vi "Data Processing for cont acq.vi"(4 "error in (no error)":errorcluster, 5 "scan parameters":T1={"scan rate\n(1000 scans/sec)"=1000.0, "scans to read\nat a time (1000)"=1000} {"scan rate\n(1000 scans/sec)" format="%.2f"}, 6 "waveform":waveform(dbl)[](array[waveform]), 7 "voltage data":sgl[][](array[numeric]) format="%.2f") -> (0 "error out":errorcluster, 1 "Intensity Graph":sgl[][](graph), 2 "processed waveform":waveform(dbl)[](array[waveform]), 3 "processed data":sgl[][](array[numeric]) format="%.2f")   [LabVIEW 2022 SP3]
doc: "My Data Processing is a subVI called by some of the analog input example VIs. These examples show you how to process and display data while an acquisition is in progress. This VI is a placeholder to show you where data processing, if any, should be done. Add whatever functions you need to its diagram. You may select Save As from the File menu to save the VI with a more meaningful name, but you should do this when all calling VIs (for example, Acquire & Process N Scans and Acquire & Proc N Scans - Trig) are open, so they are also aware of the name change. Otherwise, you must replace the subVI on each block diagram that uses the old name.\n\nThe processed data array is returned to the example VI to be displayed.\n\nError in is a cluster that indicates if an error has occurred. If so, this VI does not try to process the data, it just returns the voltage data and error unchanged. If an error occurs in your data processing, you should set the following values in the error out cluster:\n\n (bool) status: TRUE.\n\n (i32) code: the error code associated with an error.\n A value of 0 means no error, a negative value is an error,\n and a positive value is a warning.\n\n (string) source: an indication of where the \n error occurred, usually the name of the VI."
uses:
  <vilib>/Waveform/WDTOps.llb/WDT Index Channel DBL.vi
panel:
  in  "Error?":bool
  in  "Case Constant\n(See Context Help)":bool=TRUE
  in  "change window parameters ?":bool
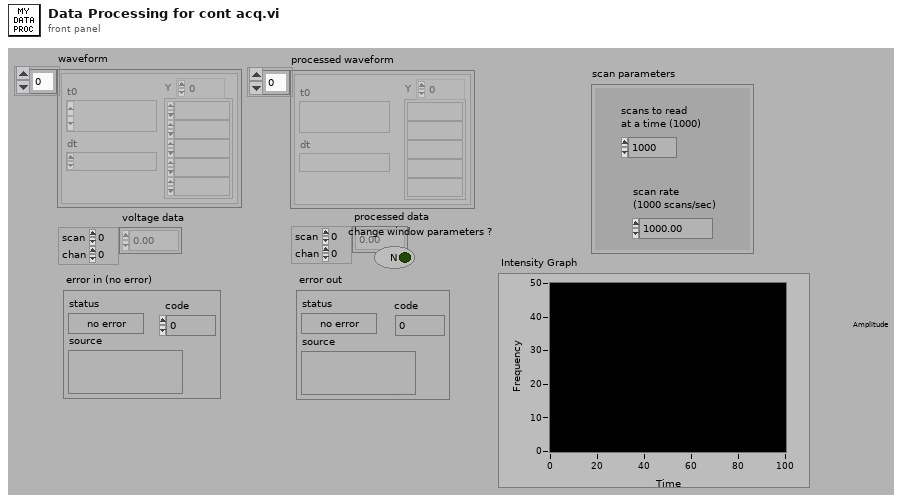
[diagram p1: front panel]
types:
  T1 = cluster{"scan rate\n(1000 scans/sec)":sgl, "scans to read\nat a time (1000)":i32}
  T2 = cluster{"scans to read\nat a time (1000)":i32, "scan rate\n(1000 scans/sec)":sgl, sgl[][]}
  T3 = cluster{"total time slices":i32, "f0":dbl, "Df":dbl, "Dt":dbl}
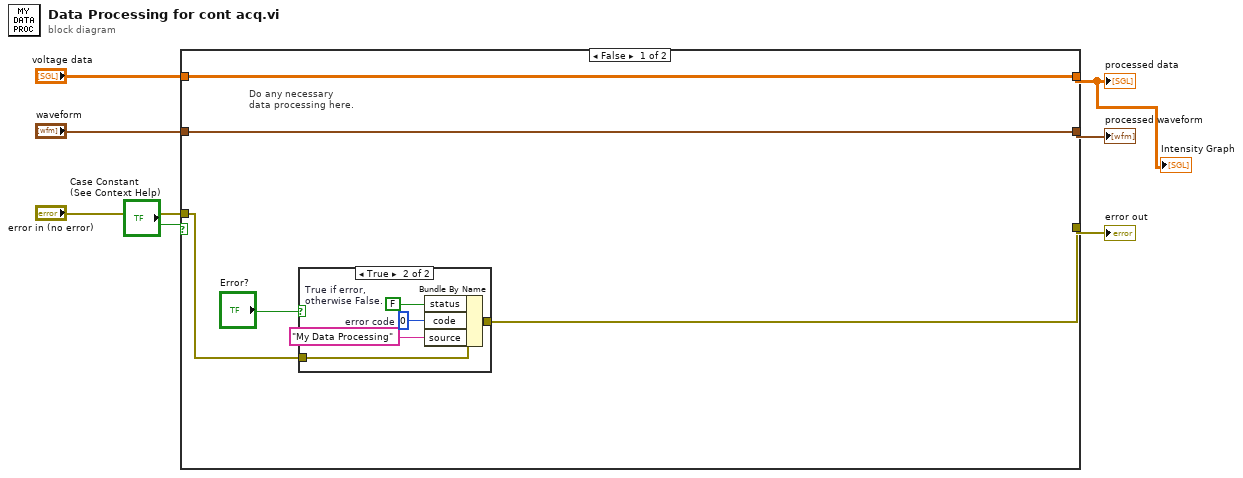
[diagram p0: block diagram]
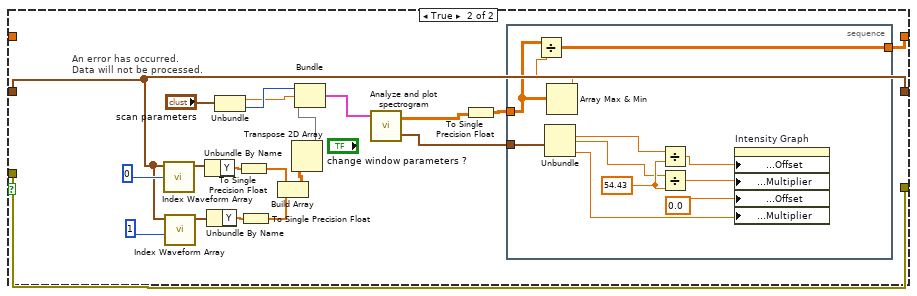
[diagram p3: hidden frame]
diagram:
  n1 = case shown="False" "Case Constant\n(See Context Help)" {
    tunnel: "error in (no error)" -> [w10 w38]
    tunnel: [w9 w38] -> w7
    tunnel: "voltage data" -> [w12 _]
    tunnel: [w12 w19] -> w3
    tunnel: "waveform" -> [w8 w27]
    tunnel: [w8 w27] -> w4
    frame False {
      # "Do any necessary\ndata processing here."
      n2 = case shown="True" "Error?" {
        tunnel: w10 -> [w13 w15]
        tunnel: [w13 w14] -> w9
        frame False {
        }
        frame True {
          w17 = 0  # error code
          w16 = FALSE  # True if error, otherwise False.
          n3 = Bundle By Name(cluster=w15, "status"=w16, "code"=w17, "source"="My Data Processing") -> (w14:errorcluster)
        }
      }
    }
    frame True {
      # "An error has occurred.\nData will not be processed."
      n4 = call-poly <vilib>:"Index Waveform Array.vi"("index"=0, "waveform array"=w27) -> ("waveform"=w37:waveform(dbl))  [unwired: 8 in, 1 out]
      n5 = call-poly <vilib>:"Index Waveform Array.vi"("index"=1, "waveform array"=w27) -> ("waveform"=w34:waveform(dbl))  [unwired: 8 in, 1 out]
      n6 = Unbundle By Name(w37) -> ("Y"=w33:dbl[])
      n7 = Unbundle By Name(w34) -> ("Y"=w32:dbl[])
      n8 = Unbundle("scan parameters") -> ("scan rate\n(1000 scans/sec)"=w23:sgl, "scans to read\nat a time (1000)"=w24:i32)
      n9 = To Single Precision Float(number=w33) -> (single precision float=w30:sgl[])
      n10 = To Single Precision Float(number=w32) -> (single precision float=w29:sgl[])
      n11 = Build Array(w30, w29) -> (w28:sgl[][])
      n12 = Transpose 2D Array(2D array=w28) -> (transposed array=w26:sgl[][])
      n13 = Bundle("scans to read\nat a time (1000)"=w24, "scan rate\n(1000 scans/sec)"=w23, w26) -> (w31:T2)  [unwired: 1 in]
      n14 = call "Analyze and plot spectrogram .vi"("datalog record"=w31) -> ("Spectrogram Plotting Parameters"=w20:T3, "Spectrogram"=w22:dbl[][])  [unwired: 2 in]
      n15 = To Single Precision Float(number=w22) -> (single precision float=w21:sgl[][])
      n16 = stacked-sequence {
        tunnel: w21 -> [w41]
        tunnel: w20 -> [w40]
        tunnel: [w39] -> w19
        frame #0 {
          w48 = 54.43 ("frequency constant")
          n17 = Unbundle(w40) -> ("f0"=w47:dbl, "Df"=w46:dbl, "Dt"=w42:dbl)  [unwired: 1 out]
          n18 = Array Max & Min(array=w41) -> (max value=w49:sgl)  [unwired: 3 out]
          n19 = Divide(x=w41, y=w49) -> (x/y=w39:sgl[][])
          n20 = Divide(x=w47, y=w48) -> (x/y=w43:dbl)
          n21 = Divide(x=w46, y=w48) -> (x/y=w44:dbl)
          n22 = property on="Intensity Graph" class="IntGraph (strict)"("Y Scale.Offset and Multiplier:Offset"=w43, "Y Scale.Offset and Multiplier:Multiplier"=w44, "X Scale.Offset and Multiplier:Offset"=0.0, "X Scale.Offset and Multiplier:Multiplier"=w42) -> ()  [unwired: 2 in, 2 out]
        }
      }
    }
  }
  "processed data" <- w3
  "error out" <- w7
  "processed waveform" <- w4
  "Intensity Graph" <- w3
